vi "GetTestItems.vi"(8 "error in (no error)":errorcluster caption="错误输入（无错误）", 11 "产品型号":refnum<vi>) -> (0 "error out":errorcluster, 4 "data":string[](array[string]))   [LabVIEW 2013]
uses:
  <vilib>/Utility/NIReport.llb/NI_report.lvclass
  SourceCode/GlobalValue.vi
  <vilib>/addons/_office/excel.llb/Excel Get Data ([str]).vi
  <vilib>/addons/_office/NI_ReportGenerationToolkit.lvlib
  <vilib>/Utility/NIReport.llb/Excel/NI_Excel.lvclass
panel:
  out "测试项目":string[][](array[string])
  out "PassYeildHistory":dbl[](array[numeric])
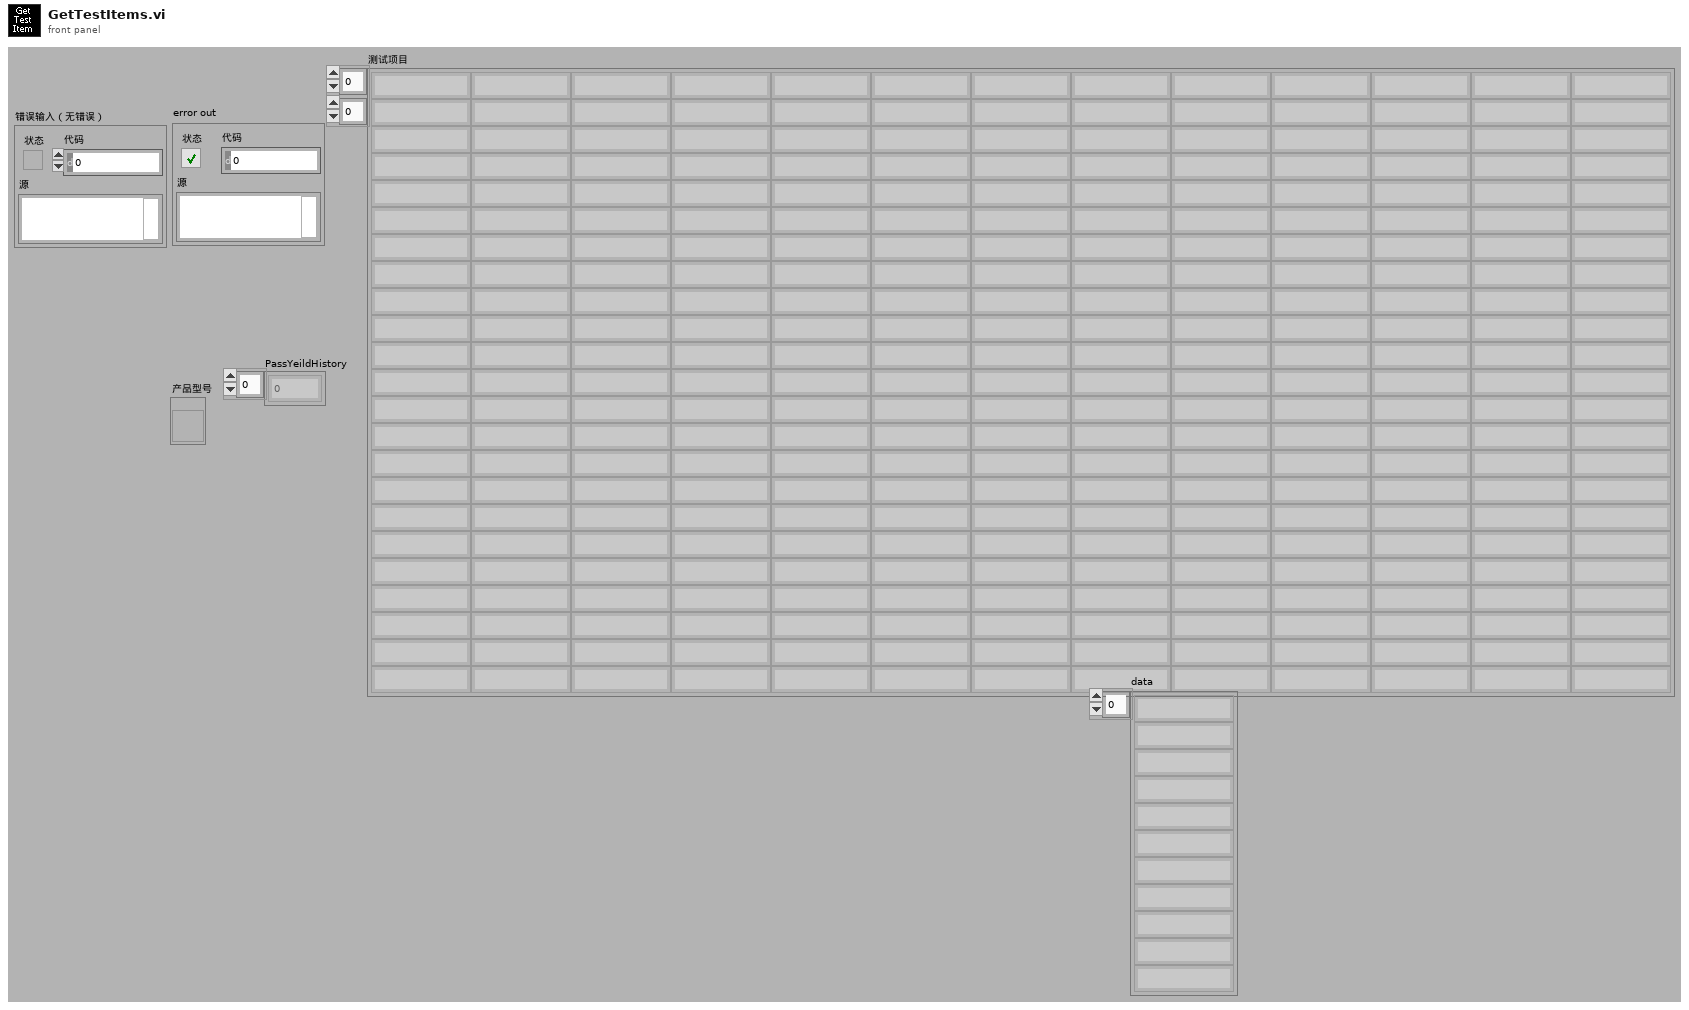
[diagram p1: front panel]
types:
  T1 = enum16{"maximized", "minimized", "normal", "no change"}
  T2 = enum16{"Standard Report", "HTML", "Word", "Excel"}
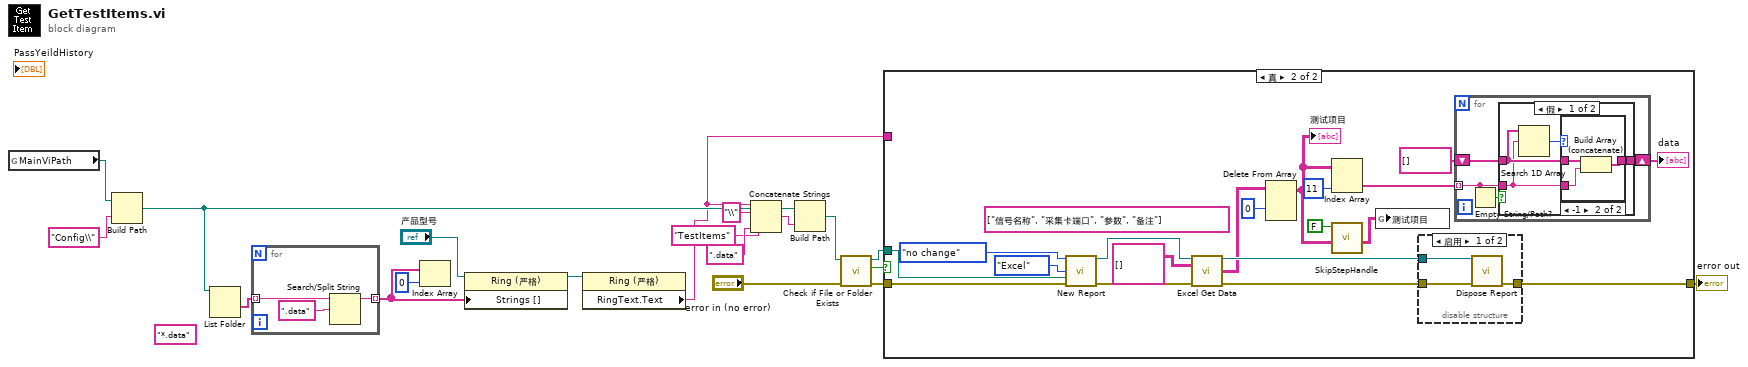
[diagram p0: block diagram]
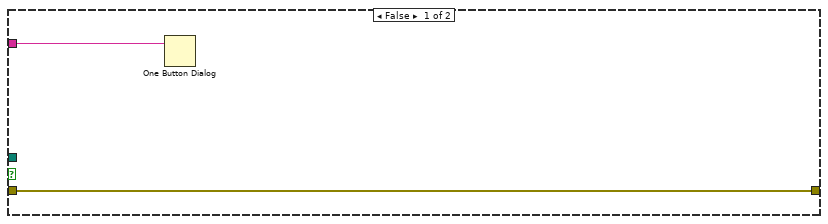
[diagram p2: hidden frame]
diagram:
  (unwired) "*.data" ("模式")
  n1 = global read "GlobalValue.vi" "MainViPath"() -> (w5:path)
  n2 = Build Path(base path=w5, name or relative path="Config\\" ("字符串")) -> (appended path=w11:path)
  n3 = List Folder(path=w11) -> (folder names=w2:string[])  [unwired: 3 in, 3 out]
  n4 = for {
    tunnel: w2 -> [w21] mode=indexing
    tunnel: [w20] -> w8 mode=indexing
    n5 = Search/Split String(string=w21, search string/char (-)=".data" ("搜索字符串/字符(-)")) -> (substring before match=w20:string)  [unwired: 3 out]
  }
  n6 = Index Array(array=w8, index=0 ("索引")) -> ()  [unwired: 1 out]
  n7 = property on="属性节点" class="Ring (严格)"(reference="产品型号", "Strings []"=w8) -> (reference out=w6:refnum<vi>)  [unwired: 1 in, 1 out]
  n8 = property on="属性节点" class="Ring (严格)"(reference=w6) -> ("RingText.Text"=w4:string)  [unwired: 1 in, 2 out]
  n9 = Concatenate Strings(w4, "\\" ("字符串"), "TestItems" ("字符串"), ".data" ("字符串")) -> (w18:string)
  n10 = Build Path(base path=w11, name or relative path=w18) -> (appended path=w15:path)
  n11 = call <vilib>:"Check if File or Folder Exists.vi"("error in (no error)"="error in (no error)", "path"=w15) -> ("error out"=w14:errorcluster, "file or folder exists?"=w17:bool, "dup path"=w16:path)  [unwired: 7 out]
  n12 = case shown="真" w17 {
    tunnel: w14 -> [w24 w42]
    tunnel: w16 -> [_ w43]
    tunnel: [w24 w40] -> w10
    tunnel: w4 -> [w23 _]
    frame False {
      n13 = One Button Dialog(message=w23) -> ()  [unwired: 1 in, 1 out]
    }
    frame True {
      (unwired) string[] ["信号名称", "采集卡端口", "参数", "备注"] ("已删除的部分")
      n14 = call <vilib>:"New Report.vi"("window state (normal)"=T1."no change", "report type"=T2."Excel", "template (empty)"=w43, "error in (no error)"=w42) -> ("report out"=w37:refnum<class "NI_report.lvclass">, "error out"=w36:errorcluster)  [unwired: 2 in, 8 out]
      n15 = call-poly <vilib>:"Excel Get Data.vi"("report in"=w37, "data type"=string[][] [], "error in (no error)"=w36) -> ("report out"=w41:refnum<class "NI_report.lvclass">, "data"=w35:string[][], "error out"=w32:errorcluster)  [unwired: 10 in]
      n16 = Delete From Array(array=w35, index (row)=0 ("索引 (行)")) -> (array with subset deleted=w29:string[][])  [unwired: 2 in, 1 out]
      "测试项目" <- w29
      n17 = Index Array(array=w29, index (col)=11 ("禁用的索引 (列)")) -> (element=w25:string[])  [unwired: 1 in]
      n18 = call "SkipStepHandle.vi"("ItemNamesIn"=w29, "ShowSkipStep?"=FALSE) -> ("ItemNamesOut"=w30:string[][])  [unwired: 9 in]
      n19 = global write "GlobalValue.vi" "测试项目"(w30) -> ()
      n20 = disable-structure shown="启用" {
        disable-tunnel: w41 -> [w59 _]
        disable-tunnel: [w58 _] -> w40
        disable-tunnel: w32 -> [w57 _]
        frame Enabled {
          n21 = call-dynamic "Dispose Report.vi"("report in"=w59, "error in (no error)"=w57) -> ("error out"=w58:errorcluster)  [unwired: 3 in, 10 out]
        }
        frame Disabled {
        }
      }
      n22 = for "For循环" {
        shift-right: [w46] -> w26
        shift-left: string[] [] -> [w47]
        tunnel: w25 -> [w45] mode=indexing
        n23 = Empty String/Path?(string/path=w45) -> (empty?=w44:bool)
        n24 = case shown="假" w44 {
          tunnel: w47 -> [w50 w56]
          tunnel: [w49 w56] -> w46
          tunnel: w45 -> [w48 _]
          frame False {
            n25 = Search 1D Array(1D array=w50, element=w48) -> (index of element=w51:i32)  [unwired: 1 in]
            n26 = case shown="-1" w51 {
              tunnel: w50 -> [w52 w54]
              tunnel: [w52 w53] -> w49
              tunnel: w48 -> [_ w55]
              frame 1, Default {
              }
              frame -1 {
                n27 = Build Array (concatenate)(w54, w55) -> (w53:string[])
              }
            }
          }
          frame True {
          }
        }
      }
      "data" <- w26
    }
  }
  "error out" <- w10
